vi "tm3samp_09_wview.vi"() -> ()   [LabVIEW 2023]
panel:
  out "Image B":u16[][](graph) caption="Image"
  out "Image A":u16[][](graph) caption="Image"
  in  "Vertical Width":i32=512
  in  "Horizontal Width":i32=1024
  in  "Vertical Offset B":i32=64
  in  "Horizontal Offset B":i32=256
  in  "Vertical Offset A":i32=128
  in  "Horizontal Offset A":i32=512
  out "Frames Per Second":dbl
  in  "Quit":bool
  out "Error Out":errorcluster {"code" format="%.0x"}
  # "This is just a simple example\nof how to setup a camera for\na W-View application with\na Flash4.0 LT"
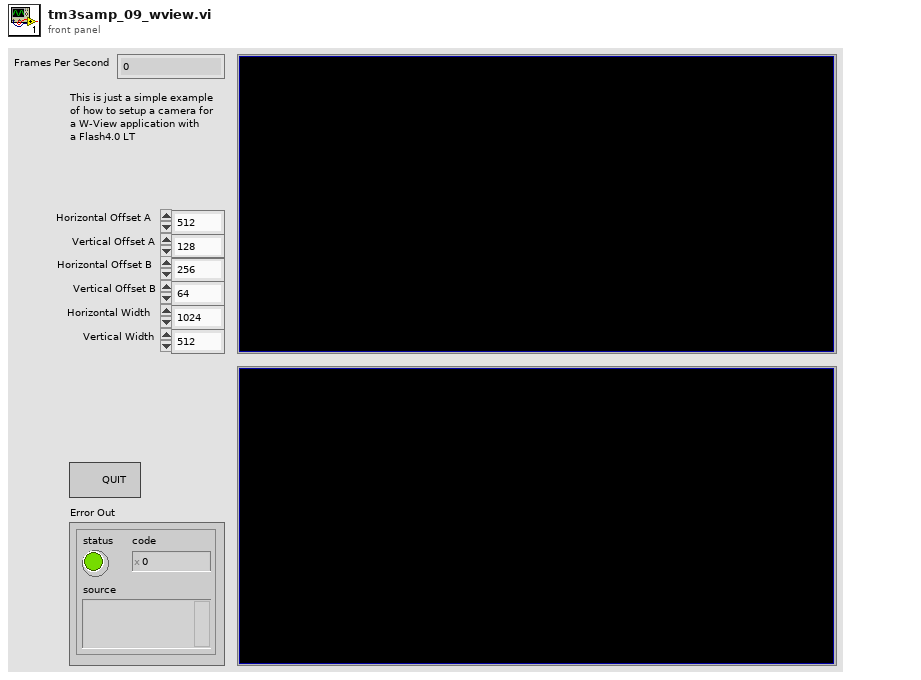
[diagram p1: front panel]
types:
  T1 = cluster{"Horizontal Offset A":i32, "Vertical Offset A":i32, "Horizontal Offset B":i32, "Vertical Offset B":i32, "Horizontal Width":i32, "Vertical Width":i32}
  T2 = cluster{"height":u32, "width":u32, "datatype":u32}
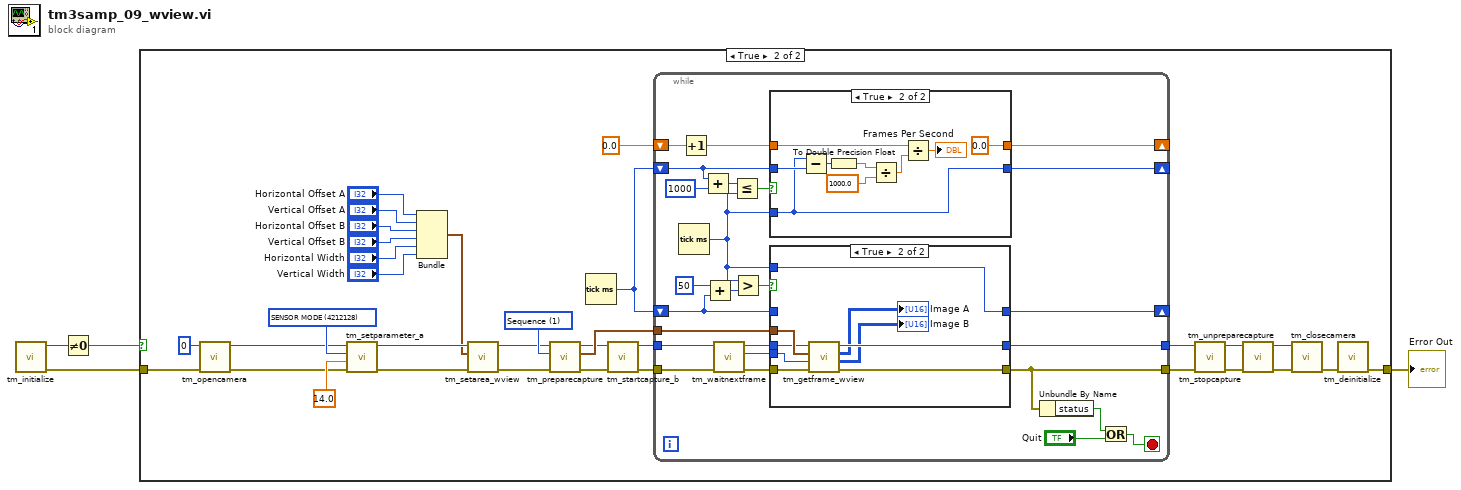
[diagram p0: block diagram]
diagram:
  n1 = call "tm_initialize.vi"() -> ("error out"=w1:errorcluster, "Number Of Cameras"=w2:u32)  [unwired: 8 in, 2 out]
  n2 = Not Equal To 0?(x=w2) -> (x != 0?=w4:bool)
  n3 = case shown="True" w4 {
    tunnel: w1 -> [w5 w38]
    tunnel: [w5 w35] -> w3
    frame False {
    }
    frame True {
      w19 = u32 4212128 items=["SENSOR MODE"=4212128, "CCD MODE"=4212384, "READOUT MODE"=4211872, "ACTIVE VIEW INDEX"=4343136, "BITS PER CHANNEL"=4342976, "IMAGE PIXEL TYPE"=4343296, "BINNING"=4215968, "EXPOSURE TIME"=2049184, "CONTRAST GAIN"=3163312, "CONTRAST OFFSET"=3163328, "LIGHT MODE"=2114720, "SENSITIVITY"=2114992, "PHOTON IMAGING MODE"=2115200, "HIGH DYNAMIC RANGE MODE"=3163360, "WHITE BALANCE"=3163568, "TEMPERATURE"=2115232, "TEMPERATURE TARGET"=2115264, "SENSOR COOLER FAN"=2115296, "LINEBUNDLE HEIGHT"=4212192, "MECHANICAL SHUTTER"=2115488, "BACK FOCUS POSITION"=8422304, "TRIGGER CONNECTOR"=1066432, "TRIGGER SOURCE"=1066144, "OUTPUT TRIGGER SOURCE"=1852576, "TRIGGER GLOBAL EXPOSURE"=2049680, "FIRST TRIGGER BEHAVIOR"=2049696, "CHANNEL SYNC"=1852352, "READOUT DIRECTION"=4211904, "PRE HSYNC COUNT"=1852704, "INTERNAL LINE SPEED"=4191408, "INTERNAL LINE INTERVAL"=4191424] ("Parameter")
      w26 = 1 items=["Snap", "Sequence"] ("Capture mode")
      n4 = call "tm_opencamera.vi"("error in (no error)"=w38, "Camera Index"=u32 0) -> ("error out"=w17:errorcluster, "Handle out"=w18:u32)  [unwired: 7 in, 1 out]
      n5 = call "tm_setparameter_a.vi"("error in (no error)"=w17, "Value in"=14.0, "Parameter"=w19, "Handle in"=w18) -> ("error out"=w15:errorcluster, "Handle out"=w16:u32)  [unwired: 6 in]
      n6 = Bundle("Horizontal Offset A"="Horizontal Offset A", "Vertical Offset A"="Vertical Offset A", "Horizontal Offset B"="Horizontal Offset B", "Vertical Offset B"="Vertical Offset B", "Horizontal Width"="Horizontal Width", "Vertical Width"="Vertical Width") -> (w12:T1)  [unwired: 1 in]
      n7 = call "tm_setarea_wview.vi"("error in (no error)"=w15, "Sub Region"=w12, "Handle in"=w16) -> ("error out"=w14:errorcluster, "Handle out"=w13:u32)  [unwired: 7 in]
      n8 = call "tm_preparecapture.vi"("error in (no error)"=w14, "Capture mode"=w26, "Handle in"=w13) -> ("error out"=w23:errorcluster, "Buffer Info"=w25:T2, "Handle out"=w24:u32)  [unwired: 5 in, 1 out]
      n9 = Tick Count (ms)() -> (millisecond timer value=w21:u32)
      n10 = call "tm_startcapture_b.vi"("error in (no error)"=w23, "Handle in"=w24) -> ("error out"=w27:errorcluster, "Handle out"=w28:u32)  [unwired: 8 in]
      n11 = while {
        tunnel: [w42] -> w31
        tunnel: [w43] -> w32
        tunnel: w25 -> [w40]
        tunnel: w28 -> [w60]
        tunnel: w27 -> [w61]
        shift-right: [w58] -> _
        shift-left: w21 -> [w55]
        shift-right: [w59] -> _
        shift-left: 0.0 -> [w52]
        shift-right: [w41] -> _
        shift-left: w21 -> [w44]
        stop <- w39 stop-if-true
        n12 = Tick Count (ms)() -> (millisecond timer value=w45:u32)
        n13 = Increment(x=w52) -> (x+1=w53:dbl)
        n14 = Add(x=w55, y=u32 1000) -> (x+y=w57:u32)
        n15 = Add(x=u32 50, y=w44) -> (x+y=w47:u32)
        n16 = call "tm_waitnextframe.vi"("error in (no error)"=w61, "Handle in"=w60) -> ("error out"=w50:errorcluster, "Frame Index"=w49:i32, "Handle out"=w51:u32)  [unwired: 6 in, 1 out]
        n17 = Less Or Equal?(x=w57, y=w45) -> (x <= y?=w54:bool)
        n18 = Greater?(x=w45, y=w47) -> (0:w46:bool)
        n19 = case shown="True" w54 {
          tunnel: w55 -> [w77 w80]
          tunnel: [w77 w78] -> w58
          tunnel: w53 -> [w76 w84]
          tunnel: w45 -> [_ w78]
          tunnel: [w76 0.0] -> w59
          frame False {
          }
          frame True {
            n20 = Subtract(x=w78, y=w80) -> (x-y=w79:u32)
            n21 = To Double Precision Float(number=w79) -> (double precision float=w86:dbl)
            n22 = Divide(x=w86, y=1000.0) -> (x/y=w83:dbl)
            n23 = Divide(x=w84, y=w83) -> (x/y=→"Frames Per Second":dbl)
          }
        }
        n24 = case shown="True" w46 {
          tunnel: w51 -> [w66 w71]
          tunnel: w50 -> [w65 w74]
          tunnel: w49 -> [_ w73]
          tunnel: w44 -> [w64 _]
          tunnel: w45 -> [_ w75]
          tunnel: [w66 w69] -> w42
          tunnel: [w65 w70] -> w43
          tunnel: [w64 w75] -> w41
          tunnel: w40 -> [_ w72]
          frame False {
          }
          frame True {
            n25 = call "tm_getframe_wview.vi"("error in (no error)"=w74, "Frame Index"=w73, "Buffer Info"=w72, "Handle in"=w71) -> ("error out"=w70:errorcluster, "Data B"=→"Image B":u16[][], "Data A"=→"Image A":u16[][], "Handle out"=w69:u32)  [unwired: 3 in, 1 out]
          }
        }
        n26 = Unbundle By Name(w43) -> ("status"=w63:bool)
        n27 = Or(x=w63, y="Quit") -> (x .or. y?=w39:bool)
      }
      n28 = call "tm_stopcapture.vi"("error in (no error)"=w32, "Handle in"=w31) -> ("error out"=w29:errorcluster, "Handle out"=w30:u32)  [unwired: 8 in]
      n29 = call "tm_unpreparecapture.vi"("error in (no error)"=w29, "Handle in"=w30) -> ("error out"=w34:errorcluster, "Handle out"=w33:u32)  [unwired: 8 in]
      n30 = call "tm_closecamera.vi"("error in (no error)"=w34, "Handle in"=w33) -> ("error out"=w36:errorcluster)  [unwired: 9 in]
      n31 = call "tm_deinitialize.vi"("error in (no error)"=w36) -> ("error out"=w35:errorcluster)  [unwired: 10 in]
    }
  }
  "Error Out" <- w3
